vi "Vision Processing.vi"(4 "error in (no error)":errorcluster, 7 "Image Size":T3=enum."320x240") -> ()   [LabVIEW 2016]
doc: "This VI runs in parallel to other tasks. It gets images from the camera, processes them for color or shape and use that information to affect robot behavior."
uses:
  <vilib>/Rock Robotics/WPI/Camera/WPI_CameraImageSize.ctl
  <vilib>/vision/Image Controls.llb/IMAQ Image.ctl
  <vilib>/Rock Robotics/WPI/Camera/WPI_CameraExposure Values.ctl
  <vilib>/Rock Robotics/WPI/Camera/WPI_CameraFrameRate.ctl
  Robot Global Data.vi
  <vilib>/vision/NI_Vision_Development_Module.lvlib
panel:
  out "Right":bool
  out "Right":dbl
  out "Left":dbl
  out "output cluster":cluster{"Yaw Angle":dbl, "Distance":dbl}
  out "Image Out":T1
  out "frequency":dbl
  out "Detected and good":bool
  out "Particle Reports (Pixels)":T2(array[cluster]) {"Orientation" format="%.2f"; "Dimensions"."Height" format="%.2f"; "Dimensions"."Width" format="%.2f"; "Center of Mass"."Y" format="%.2f"; "Center of Mass"."X" format="%.2f"; "Bounding Rect"."Bottom" format="%.2f"; "Bounding Rect"."Right" format="%.2f"; "Bounding Rect"."Top" format="%.2f"; "Bounding Rect"."Left" format="%.2f"; "Number of Holes" format="%.2f"; "Area" format="%.2f"}
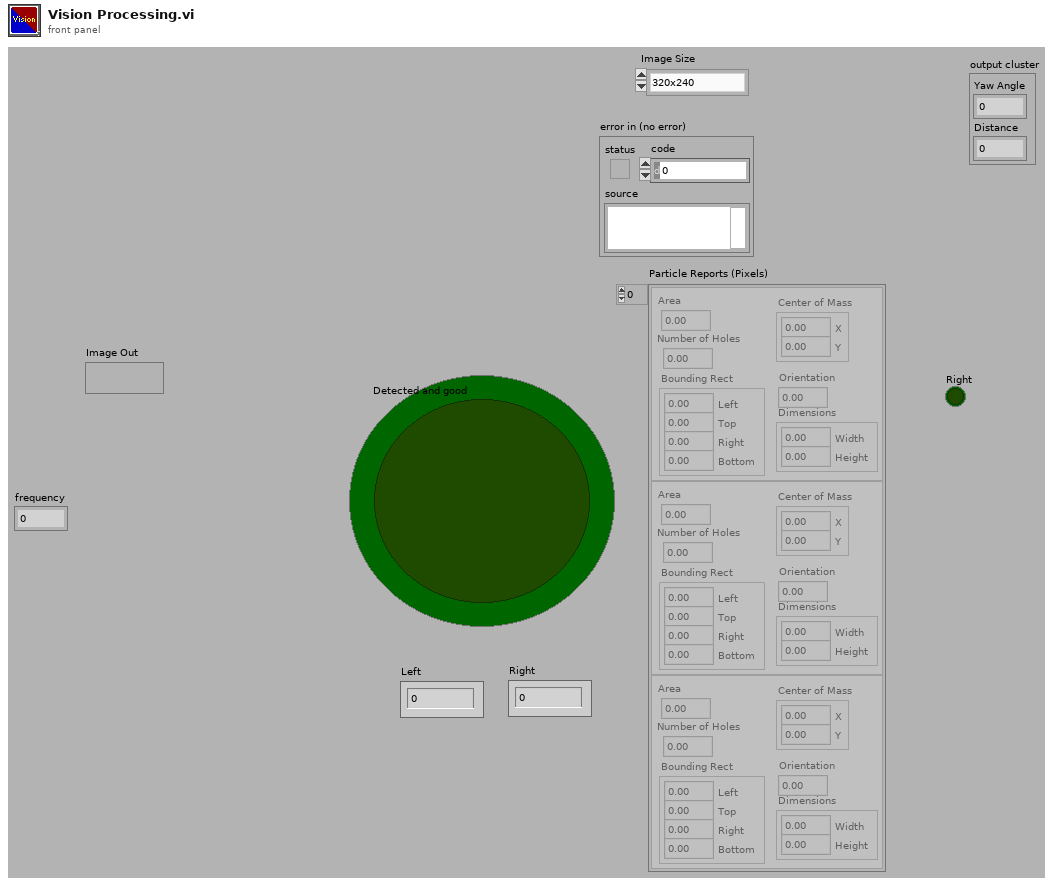
[diagram p1: front panel]
types:
  T1 = typedef "IMAQ Image.ctl" = refnum<image>
  T2 = cluster{"Area":dbl, "Number of Holes":dbl, "Bounding Rect":cluster{"Left":dbl, "Top":dbl, "Right":dbl, "Bottom":dbl}, "Center of Mass":cluster{"X":dbl, "Y":dbl}, "Orientation":dbl, "Dimensions":cluster{"Width":dbl, "Height":dbl}}[]
  T3 = typedef "WPI_CameraImageSize.ctl" = enum16{"640x480", "320x240", "160x120", "Custom"}
  T4 = typedef "WPI_CameraFrameRate.ctl" = u32
  T5 = typedef "WPI_CameraExposure Values.ctl" = enum16{"Auto", "Flicker-free 50 Hz", "Flicker-free 60 Hz", "Hold current", "Custom"}
  T6 = typedef "Image Type" = u32
  T7 = typedef "WPI_CameraDevRef.ctl" = cluster{"Camera Address":string, "CameraStatus":errorcluster}
  T8 = cluster{"Yaw":dbl, "Roll":dbl, "Pitch":dbl, "Heading":dbl, "Fused Heading":dbl}
  T9 = cluster{"Area":dbl, "Number of Holes":dbl, "Bounding Rect":cluster{"Left":dbl, "Top":dbl, "Right":dbl, "Bottom":dbl}, "Center of Mass":cluster{"X":dbl, "Y":dbl}, "Orientation":dbl, "Dimensions":cluster{"Width":dbl, "Height":dbl}}
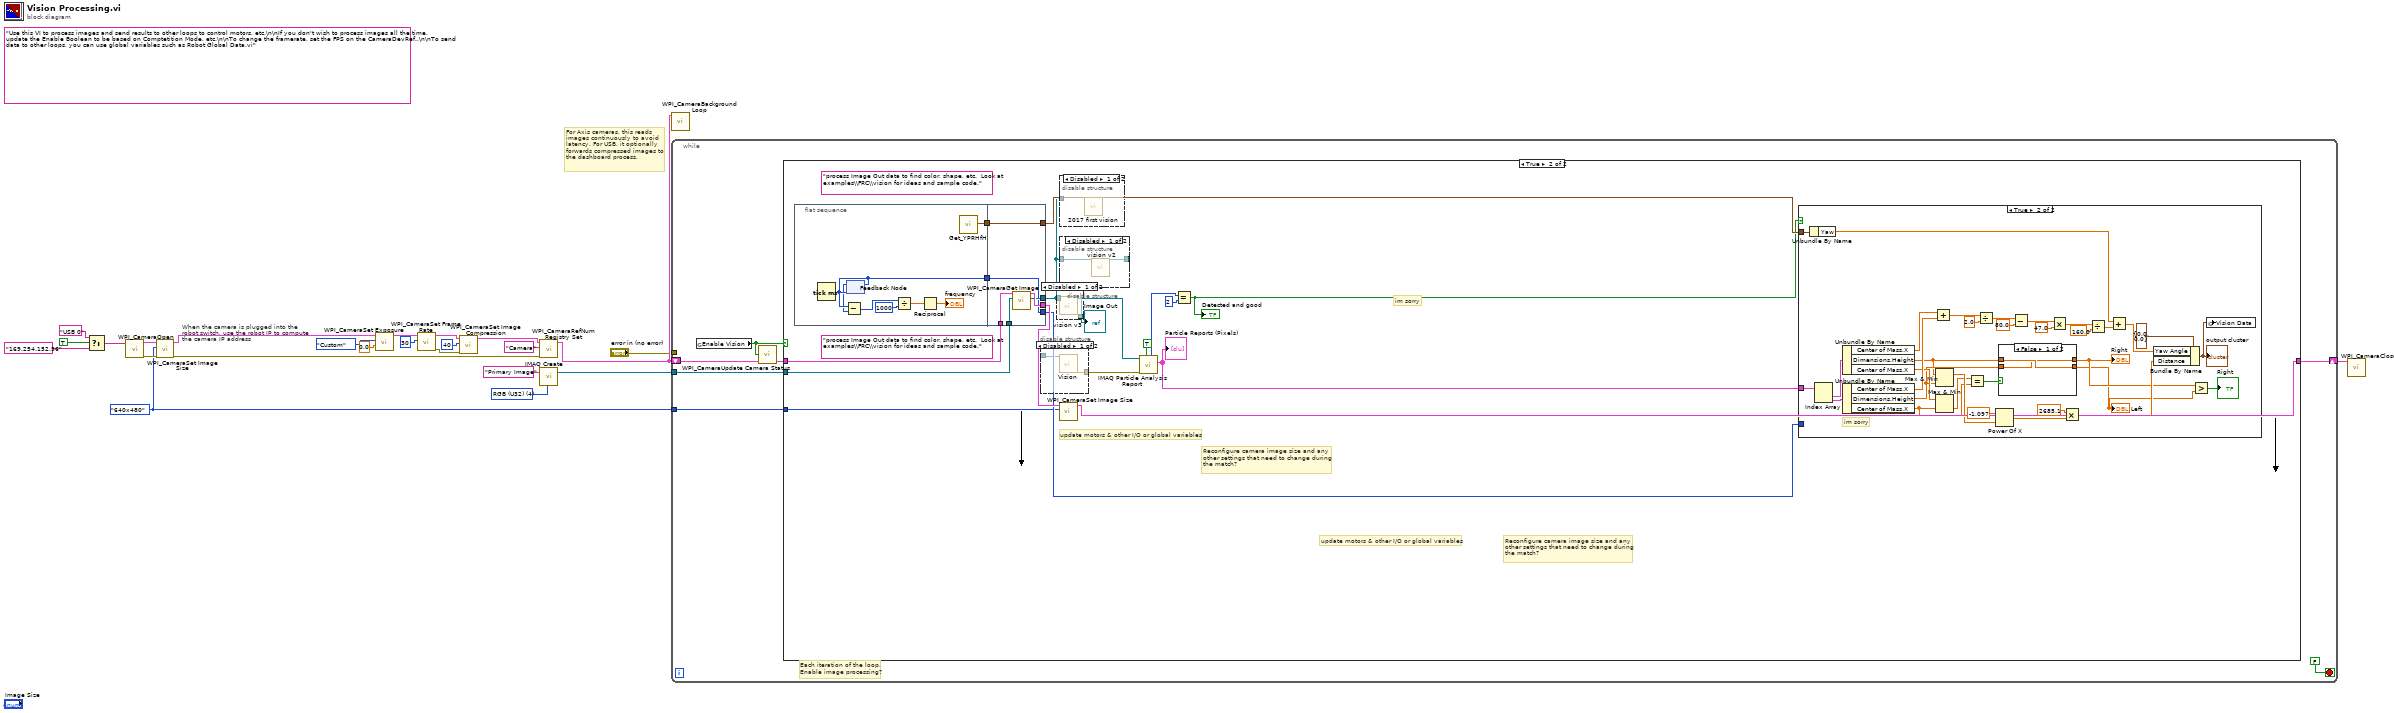
[diagram p0: block diagram]
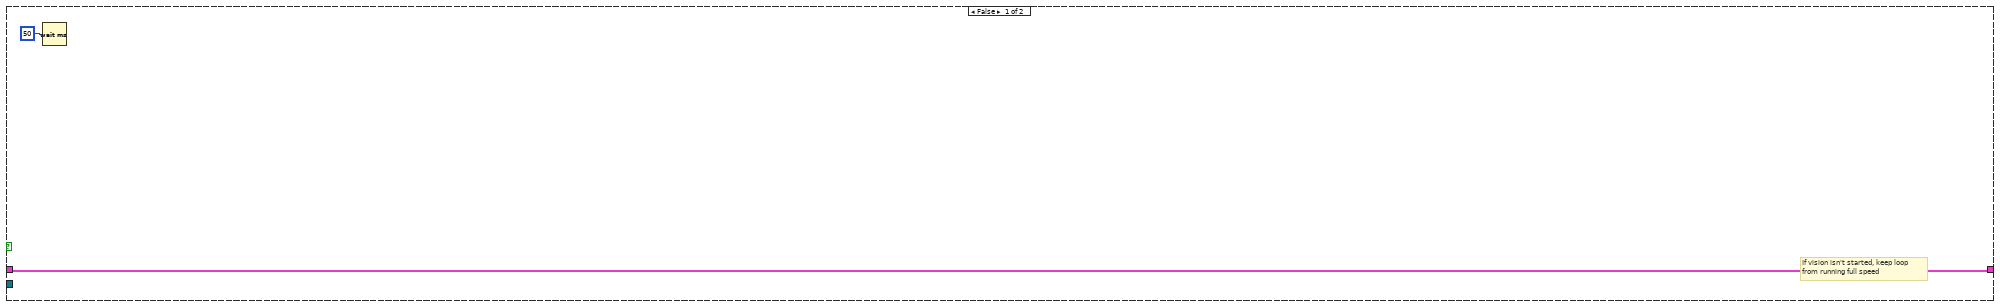
[diagram p2: hidden frame]
diagram:
  w1 = WPI_CameraImageSize."640x480" ("Image Size")
  (unwired) "Use this VI to process images and send results to other loops to control motors, etc.\n\nIf you don't wish to process images all the time, update the Enable Boolean to be based on Comptetition Mode, etc.\n\nTo change the framerate, set the FPS on the CameraDevRef..\n\nTo send data to other loops, you can use global variables such as Robot Global Data.vi"
  w24 = T6 4 items=["Grayscale (U8)", "Grayscale (I16)", "Grayscale (SGL)", "Complex (CSG)", "RGB (U32)", "HSL (U32)", "RGB (U64)"] ("Image Type")
  # "When the camera is plugged into the\nrobot switch, use the robot IP to compute\nthe camera IP address"
  # "For Axis cameras, this reads\nimages continuously to avoid\nlatency. For USB, it optionally\nforwards compressed images to\nthe dashboard process."
  n1 = Select(t="USB 0" ("format string"), s=TRUE ("dot notation? (F)"), f="169.254.152.96" ("format string")) -> (s? t:f=w13:string)
  n2 = call <vilib>:"WPI_CameraOpen.vi"("Camera Address"=w13) -> ("error out"=w19:errorcluster, "CameraDevRef"=w20:T7)  [unwired: 1 in, 8 out]
  n3 = call <vilib>:"WPI_CameraSet Image Size.vi"("error in (no error)"=w19, "Image Size"=w1, "CameraDevRef"=w20) -> ("error out"=w11:errorcluster, "CameraDevRef Out"=w10:T7)  [unwired: 1 in, 6 out]
  n4 = call <vilib>:"WPI_CameraSet Exposure.vi"("Exposure (%)"=0.0, "Exposure"=WPI_CameraExposure_Values."Custom", "CameraDevRef"=w10) -> ("CameraDevRef Out"=w3:T7)  [unwired: 7 in, 1 out]
  n5 = call <vilib>:"WPI_CameraSet Frame Rate.vi"("Frame Rate (fps)"=T4 30, "CameraDevRef"=w3) -> ("error out"=w6:errorcluster, "CameraDevRef Out"=w5:T7)  [unwired: 8 in]
  n6 = call <vilib>:"WPI_CameraSet Image Compression.vi"("error in (no error)"=w6, "Compression"=40, "CameraDevRef"=w5) -> ("CameraDevRef Out"=w2:T7)  [unwired: 7 in, 1 out]
  n7 = call <vilib>:"WPI_CameraRefNum Registry Set.vi"("error in (no error)"=w11, "refnum name"="Camera", "CameraDevRef"=w2) -> ("CameraDevRef"=w18:T7)  [unwired: 1 in, 7 out]
  n8 = call "IMAQ Create"("Image Name"="Primary Image", "Image Type"=w24) -> ("New Image"=w22:T1)  [unwired: 2 in, 2 out]
  n9 = call <vilib>:"WPI_CameraBackground Loop.vi"("CameraDevRef"=w18) -> ()  [unwired: 11 in]
  n10 = while {
    shift-right: [w30] -> w17
    shift-left: w18 -> [w28]
    tunnel: w22 -> [w29]
    tunnel: "error in (no error)" -> [_]
    tunnel: w1 -> [w25]
    stop <- FALSE stop-if-true
    # "Each iteration of the loop,\nEnable image processing?"
    n11 = global read "Robot Global Data.vi" "Enable Vision"() -> (w26:bool)
    n12 = call <vilib>:"WPI_CameraUpdate Camera Status.vi"("CameraDevRef In"=w28, "Enable Vision"=w26) -> ("CameraDevRef Out"=w27:T7)  [unwired: 3 in]
    n13 = case shown="True" w26 {
      tunnel: w29 -> [_ w50]
      tunnel: [w33 w48] -> w30
      tunnel: w27 -> [w33 w49]
      tunnel: w25 -> [_ w38]
      frame False {
        # "If vision isn't started, keep loop\nfrom running full speed"
        n14 = Wait (ms)(milliseconds to wait=u32 50) -> ()  [unwired: 1 out]
      }
      frame True {
        (unwired) "process Image Out data to find color, shape, etc.  Look at examples\\FRC\\vision for ideas and sample code."
        (unwired) "process Image Out data to find color, shape, etc.  Look at examples\\FRC\\vision for ideas and sample code."
        # "im sorry"
        # "update motors & other I/O or global variables"
        # "Reconfigure camera image size and any\nother settings that need to change during\nthe match?"
        # "update motors & other I/O or global variables"
        # "Reconfigure camera image size and any\nother settings that need to change during\nthe match?"
        n15 = flat-sequence {
          tunnel: [w60] -> w47
          tunnel: [w58] -> w46
          tunnel: [w70] -> w45
          tunnel: [w69] -> w36
          tunnel: [w68] -> w42
          tunnel: w47 -> [w68]
          tunnel: [w67] -> w41
          tunnel: w46 -> [w67]
          tunnel: w49 -> [w66]
          tunnel: w50 -> [w65]
          frame #0 {
            n16 = Tick Count (ms)() -> (millisecond timer value=w60:u32)
            n17 = feedback-in #1(w60) -> ()
            n18 = feedback #1(w60) -> (w59:u32)
            n19 = Subtract(x=w60, y=w59) -> (x-y=w64:u32)
            n20 = Divide(x=w64, y=u32 1000) -> (x/y=w62:dbl)
            n21 = Reciprocal(x=w62) -> (1/x=→"frequency":dbl)
            n22 = call <vilib>:"Get_YPRHfH.vi"() -> ("YRPHfH"=w58:T8)  [unwired: 11 in]
          }
          frame #1 {
            n23 = call <vilib>:"WPI_CameraGet Image.vi"("Image"=w65, "CameraDevRef"=w66) -> ("Image Out"=w69:T1, "CameraDevRef Out"=w70:T7)  [unwired: 1 in, 7 out]
          }
        }
        n24 = disable-structure shown="Disabled" {
          disable-tunnel: [w57 _] -> w44
          disable-tunnel: _ -> [w56 _]
          frame Disabled {
            n25 = call "Vision.vi"("Image In"=w56) -> ("error out"=w57:errorcluster)  [unwired: 23 in, 3 out]
          }
          frame Enabled {
          }
        }
        n26 = disable-structure shown="Disabled" {
          disable-tunnel: w36 -> [w52 _]
          disable-tunnel: [w51 _] -> w35
          frame Disabled {
            n27 = call "vision v3.vi"("Image In"=w52) -> ("Image Out"=w51:T1)  [unwired: 25 in, 1 out]
          }
          frame Enabled {
          }
        }
        "Image Out" <- w35
        n28 = disable-structure shown="Disabled" {
          disable-tunnel: w36 -> [w55 _]
          frame Disabled {
            n29 = call "2017 first vision.vi"("Image In"=w55) -> ()  [unwired: 23 in, 4 out]
          }
          frame Enabled {
          }
        }
        n30 = disable-structure shown="Disabled" {
          disable-tunnel: [w54 _] -> _
          disable-tunnel: w36 -> [w53 _]
          frame Disabled {
            n31 = call "vision v2.vi"("Image In"=w53) -> ("Image Out"=w54:T1)  [unwired: 25 in, 1 out]
          }
          frame Enabled {
          }
        }
        n32 = call <vilib>:"WPI_CameraSet Image Size.vi"("Image Size"=w38, "CameraDevRef"=w45) -> ("CameraDevRef Out"=w48:T7)  [unwired: 2 in, 7 out]
        n33 = call "IMAQ Particle Analysis Report"("Connectivity 4/8 (8)"=TRUE, "error in (no error)"=w44, "Image"=w35) -> ("Particle Reports (Pixels)"=w37:T2, "Number of Particles"=w40:i32)  [unwired: 3 in, 4 out]
        "Particle Reports (Pixels)" <- w37
        n34 = Equal?(x=w40, y=2) -> (x = y?=w34:bool)
        "Detected and good" <- w34
        n35 = case shown="True" w34 {
          tunnel: w37 -> [_ w103]
          tunnel: w42 -> [_ _]
          tunnel: w41 -> [_ w92]
          frame False {
          }
          frame True {
            # "im sorry"
            n36 = Unbundle By Name(w92) -> ("Yaw"=w91:dbl)
            n37 = Index Array(array=w103) -> (element #1=w102:T9, element #2=w101:T9)  [unwired: 2 in]
            n38 = Unbundle By Name(w102) -> ("Center of Mass.X"=w100:dbl, "Dimensions.Height"=w74:dbl, "Center of Mass.X"=w79:dbl)
            n39 = Unbundle By Name(w101) -> ("Center of Mass.X"=w99:dbl, "Dimensions.Height"=w75:dbl, "Center of Mass.X"=w77:dbl)
            n40 = Add(x=w100, y=w99) -> (x+y=w98:dbl)
            n41 = Max & Min(x=w74, y=w75) -> (max(x,y)=w80:dbl)  [unwired: 1 out]
            n42 = Max & Min(x=w79, y=w77) -> (min(x,y)=w78:dbl)  [unwired: 1 out]
            n43 = Equal?(x=w78, y=w77) -> (x = y?=w76:bool)
            n44 = Divide(x=w98, y=2.0) -> (x/y=w96:dbl)
            n45 = Power Of X(1:w80, 2:-1.097 ("x")) -> (0:w84:dbl)
            n46 = case shown="False" w76 {
              tunnel: w75 -> [w104 w107]
              tunnel: [w105 w107] -> w72
              tunnel: w74 -> [w105 w106]
              tunnel: [w104 w106] -> w73
              frame False {
              }
              frame True {
              }
            }
            "Left" <- w72
            "Right" <- w73
            n47 = Subtract(x=w96, y=80.0) -> (x-y=w94:dbl)
            n48 = Multiply(x=w94, y=47.0) -> (x*y=w87:dbl)
            n49 = Multiply(x=2685.1, y=w84) -> (x*y=w82:dbl)
            n50 = Divide(x=w87, y=160.0) -> (x/y=w89:dbl)
            n51 = Add(x=w91, y=w89) -> (x+y=w90:dbl)
            n52 = Bundle By Name(cluster=cluster{"Yaw Angle":dbl, "Distance":dbl} {"Yaw Angle"=0.0, "Distance"=0.0} ("Vision Data"), "Yaw Angle"=w90, "Distance"=w82) -> (w85:cluster{"Yaw Angle":dbl, "Distance":dbl})
            "output cluster" <- w85
            n53 = Greater?(x=w73, y=w72) -> (0:→"Right":bool)
            n54 = global write "Robot Global Data.vi" "Vision Data"(w85) -> ()
          }
        }
      }
    }
  }
  n55 = call <vilib>:"WPI_CameraClose.vi"("CameraDevRef"=w17) -> ()  [unwired: 1 in, 10 out]
